vi "Write Sense_Point.vi"(8 "error in":errorcluster, 10 "Sense Point":T1, 11 "36234A in":refnum<class "36234A.lvclass">) -> (0 "error out":errorcluster, 3 "36234A out":refnum<class "36234A.lvclass">)   [LabVIEW 2019, in "36234A.lvlib" / "36234A.lvclass"]
uses:
  Library/36234A.lvclass
  C:/Users/Public/Documents/Development/builds/Engine/Monitored Actor.lvlibp/Monitored Actor/Monitored Actor/Monitored Actor.lvclass
  builds/Instruments/PowerSupply.lvlibp/Custom Controls/Sense Point.ctl
  builds/Engine/Monitored Actor.lvlibp/Monitored Actor/Monitored Actor/Read Actor Label.vi
  builds/Instruments/PowerSupply.lvlibp/Library/PowerSupply.lvclass
  <vilib>/ErrorRing/Error Ring.xnode
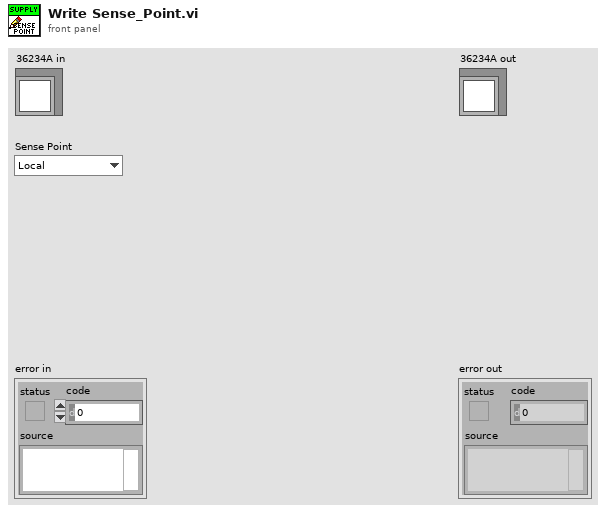
[diagram p1: front panel]
types:
  T1 = typedef "PowerSupply.lvlibp/PowerSupply.lvclass/Sense Point.ctl" = enum16{"Local", "Remote"}
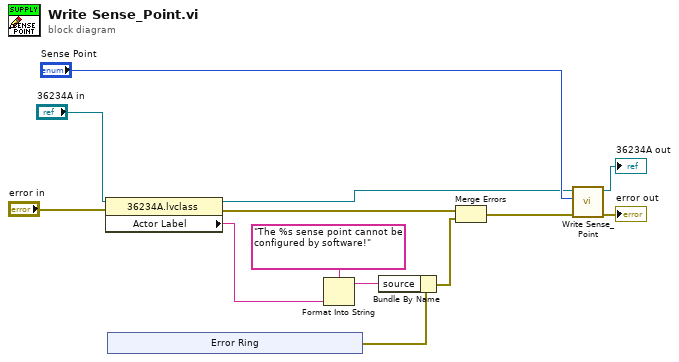
[diagram p0: block diagram]
diagram:
  n1 = property class="36234A.lvclass"(reference="36234A in", error in="error in") -> (reference out=w5:refnum<class "36234A.lvclass">, error out=w9:errorcluster, "Actor Label"=w10:string)
  n2 = xnode "Error Ring"() -> ("error out"=w6:errorcluster)
  n3 = Format Into String(format string="The %s sense point cannot be configured by software!", w10) -> (resulting string=w7:string)  [unwired: 2 in, 1 out]
  n4 = Bundle By Name(cluster=w6, "source"=w7) -> (w2:errorcluster)
  n5 = Merge Errors(w9, w2) -> (w1:errorcluster)
  n6 = call-parent "Write Sense_Point.vi"("error in"=w1, "Sense Point"="Sense Point", "PowerSupply in"=w5) -> ("error out"=→"error out":errorcluster, "PowerSupply out"=→"36234A out":refnum<class "36234A.lvclass">)  [unwired: 7 in]
